vi "GetMapTbl.vi"(2 "FalseColorDatByCH":cluster{dbl, dbl}[](array[cluster]), 3 "VarRangeMin":dbl, 4 "VarRangeMax":dbl) -> (1 "CHFalseMapTbl":T1)   [LabVIEW 2016]
panel:
  # "Description:      This VI is to get  a  false color  mapping table by channel (R/G/B)  given real var range(max/min) that you  want to map.\n\nAuthor:               L.F.Hwang  (Email: cn_gd@126.com)\n\nLast Updated:   2007/12/25"
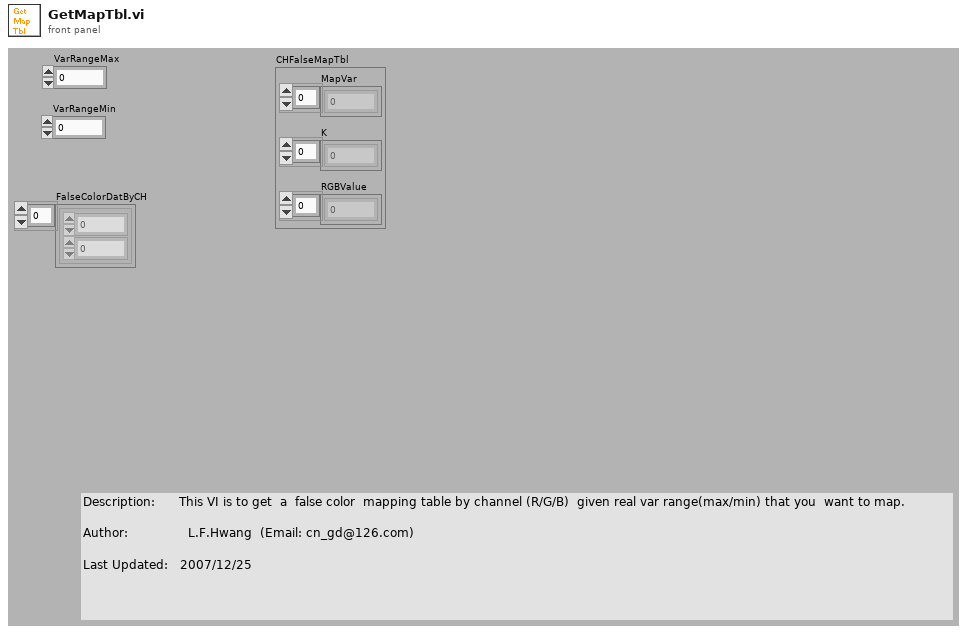
[diagram p1: front panel]
types:
  T1 = cluster{"MapVar":dbl[], "K":dbl[], "RGBValue":u8[]}
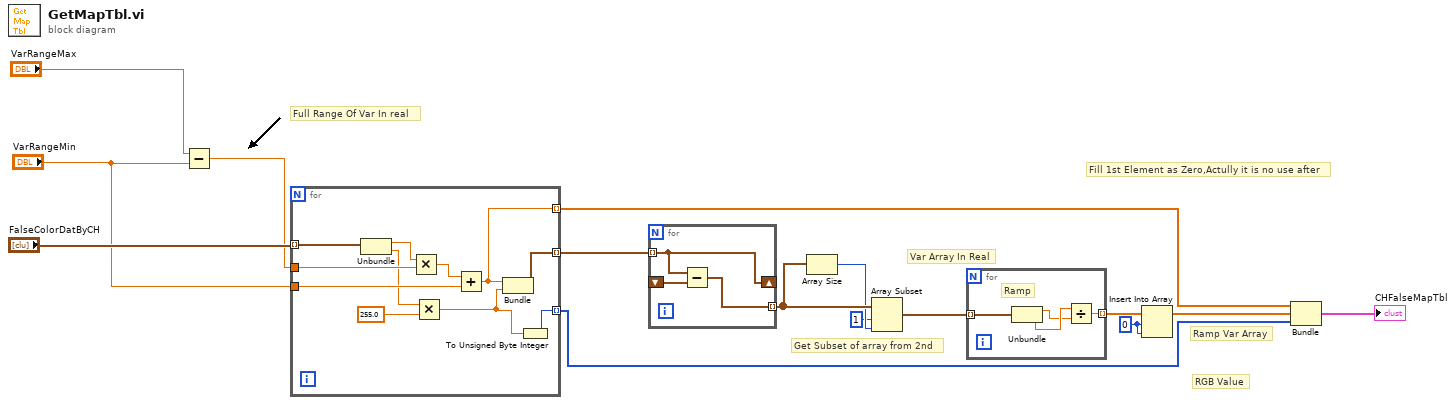
[diagram p0: block diagram]
diagram:
  w12 = 0 ("索引")
  # "RGB Value"
  # "Get Subset of array from 2nd"
  # "Var Array In Real"
  # "Fill 1st Element as Zero,Actully it is no use after"
  # "Ramp Var Array"
  # "Full Range Of Var In real"
  n1 = Subtract(x="VarRangeMax", y="VarRangeMin") -> (x-y=w6:dbl)
  n2 = for {
    tunnel: "FalseColorDatByCH" -> [w26] mode=indexing
    tunnel: w6 -> [w24]
    tunnel: "VarRangeMin" -> [w23]
    tunnel: [w21] -> w14 mode=indexing
    tunnel: [w20] -> w3 mode=indexing
    tunnel: [w16] -> w1 mode=indexing
    n3 = Unbundle(w26) -> (w25:dbl, w18:dbl)
    n4 = Multiply(x=w25, y=w24) -> (x*y=w22:dbl)
    n5 = Multiply(x=w18, y=255.0) -> (x*y=w17:dbl)
    n6 = Add(x=w22, y=w23) -> (x+y=w20:dbl)
    n7 = Bundle(w20, w17) -> (w21:cluster{dbl, dbl})  [unwired: 1 out]
    n8 = To Unsigned Byte Integer(number=w17) -> (unsigned 8bit integer=w16:u8)
  }
  n9 = for {
    tunnel: w14 -> [w29] mode=indexing
    shift-right: [w29] -> _
    shift-left: _ -> [w28]
    tunnel: [w27] -> w15 mode=indexing
    n10 = Subtract(x=w29, y=w28) -> (x-y=w27:cluster{dbl, dbl})
  }
  n11 = Array Size(array=w15) -> (size(s)=w10:i32)
  n12 = Array Subset(array=w15, index=1 ("索引"), length=w10) -> (w11:cluster{dbl, dbl}[])
  n13 = for {
    tunnel: w11 -> [w33] mode=indexing
    tunnel: [w30] -> w13 mode=indexing
    # "Ramp"
    n14 = Unbundle(w33) -> (w31:dbl, w32:dbl)
    n15 = Divide(x=w32, y=w31) -> (x/y=w30:dbl)
  }
  n16 = Insert Into Array(array=w13, index=w12, new element=w12) -> (w2:dbl[])
  n17 = Bundle(w3, w2, w1) -> (→"CHFalseMapTbl":cluster{dbl[], dbl[], u8[]})  [unwired: 1 out]
